vi "IsNull.vi"(4 "IDisposable":refnum<class "IDisposable.lvclass">) -> (1 "isNull":bool=TRUE)   [LabVIEW 2020, in "IDisposable.lvclass"]
uses:
  IDisposable.lvclass
panel:
  out "error out":errorcluster
  in  "error in (no error)":errorcluster
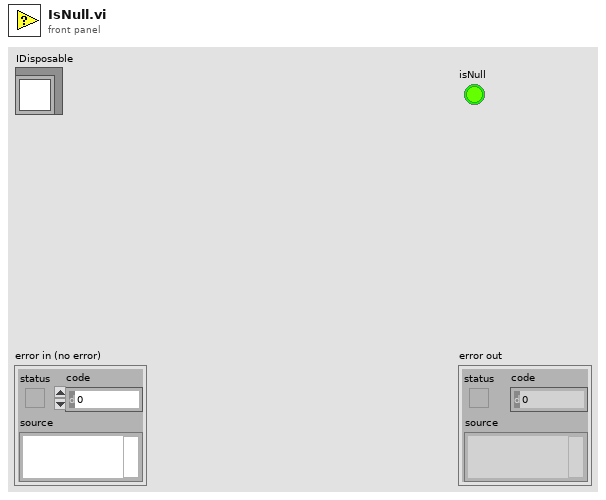
[diagram p1: front panel]
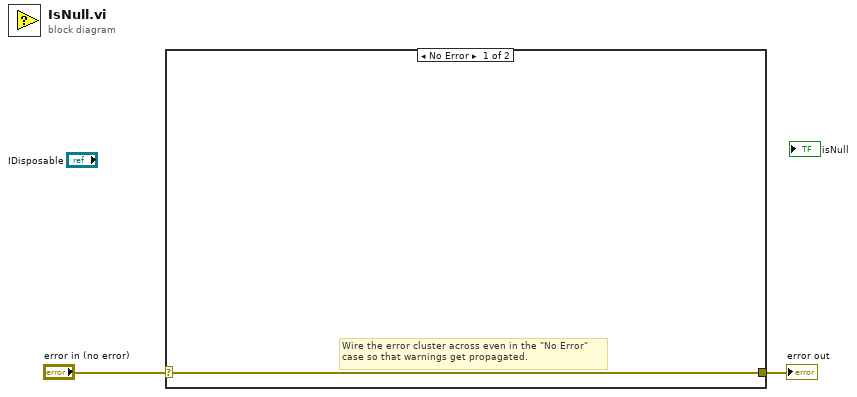
[diagram p0: block diagram]
diagram:
  n1 = case shown="No Error" "error in (no error)" {
    selector: "error in (no error)" -> [w3 w4]
    tunnel: [w3 w4] -> w1
    frame No Error {
      # "Wire the error cluster across even in the \"No Error\"\ncase so that warnings get propagated."
    }
    frame Error {
    }
  }
  "error out" <- w1
